vi "Read lambda.vi"(8 "error in (no error)":errorcluster, 11 "CRDS Cell in":refnum<class "CRDS Cell.lvclass">) -> (0 "error out":errorcluster, 2 "lambda":sgl, 3 "CRDS Cell out":refnum<class "CRDS Cell.lvclass">)   [LabVIEW 2015, in "CRDS Cell.lvclass"]
uses:
  CRDS Cell.lvclass
  CRDS Cell.lvclass/CRDS Cell.ctl
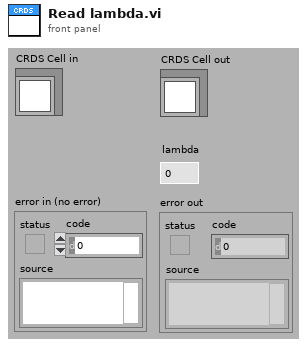
[diagram p1: front panel]
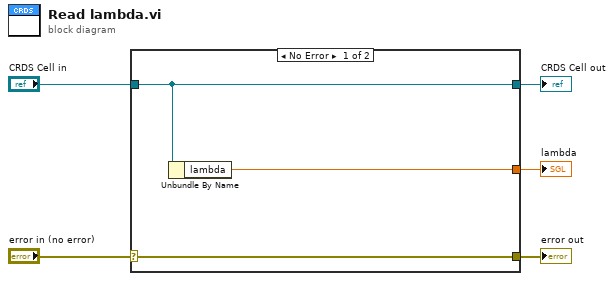
[diagram p0: block diagram]
diagram:
  n1 = case shown="No Error" "error in (no error)" {
    selector: "error in (no error)" -> [w8 w9]
    tunnel: [w8 w9] -> w4
    tunnel: [w7 w10] -> w2
    tunnel: "CRDS Cell in" -> [w7 w10]
    tunnel: [w6 _] -> w1
    frame No Error {
      n2 = Unbundle By Name(w7) -> ("lambda"=w6:dbl)
    }
    frame Error {
    }
  }
  "error out" <- w4
  "CRDS Cell out" <- w2
  "lambda" <- w1
